vi "CleanUp.vi"(0 "object in":refnum<class "CetoniPump.lvclass">, 5 "error in (no error)":errorcluster) -> (14 "object out":refnum<class "CetoniPump.lvclass">, 19 "error out":errorcluster)   [LabVIEW 2021, in "CetoniPump.lvclass"]
uses:
  CetoniPump.lvclass
  CetoniPump.lvclass/CetoniPump.ctl
  Users/olaja/AppData/Local/CETONI_SDK/lib/labview/labbCAN_Bus_API/labbCAN_Bus_API.lvlib
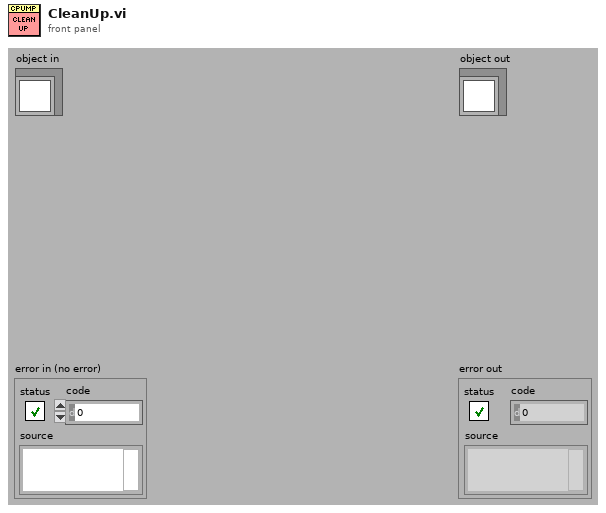
[diagram p1: front panel]
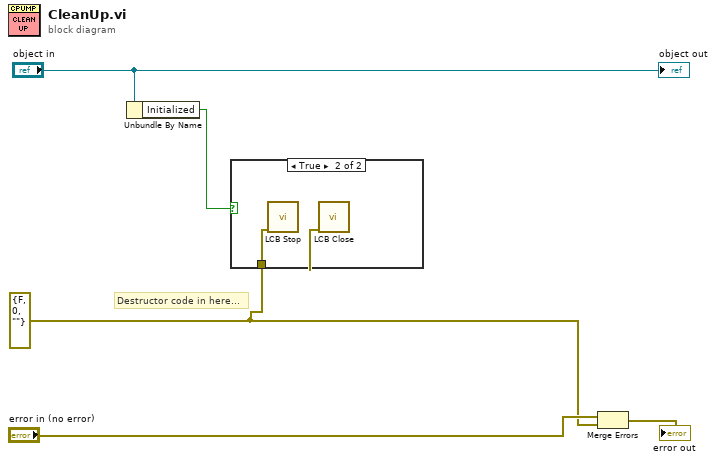
[diagram p0: block diagram]
diagram:
  w2 = errorcluster {"status"=FALSE, "code"=0, "source"=""} ("error in (no error)")
  # "Destructor code in here..."
  n1 = Unbundle By Name("object in") -> ("Initialized"=w1:bool)
  n2 = case shown="True" w1 {
    tunnel: w2 -> [_ w6]
    frame False {
    }
    frame True {
      n3 = call "LCB Stop.vi"("error in (no error)"=w6) -> ()  [unwired: 10 in, 1 out]
      n4 = call "LCB Close.vi"("error in (no error)"=w6) -> ()  [unwired: 10 in, 1 out]
    }
  }
  n5 = Merge Errors("error in (no error)", w2) -> (→"error out":errorcluster)
  "object out" <- "object in"
